vi "TextControlledInstrumCommandsToArray.vi"   [LabVIEW 2020]
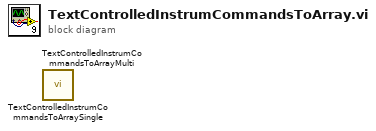
[diagram p0: block diagram]
diagram:
  n1 = call "TextControlledInstrumCommandsToArraySingle.vi"() -> ()  [unwired: 10 in, 2 out]
  n2 = call "TextControlledInstrumCommandsToArrayMulti.vi"() -> ()  [unwired: 10 in, 2 out]
